vi "DHE_DRV_set_expdelay.vi"(7 "delay(ms)":sgl, 11 "error in (no error)":errorcluster) -> (15 "error out":errorcluster)   [LabVIEW 2016]
doc: "This VI closes the I/O interface with the instrument."
uses:
  c/lib/libarcDHE.so
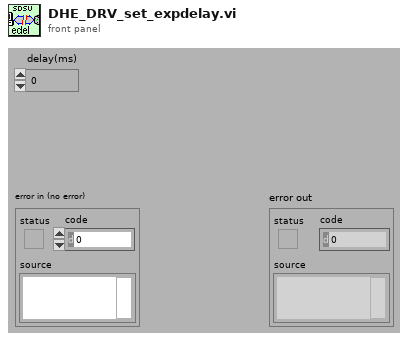
[diagram p1: front panel]
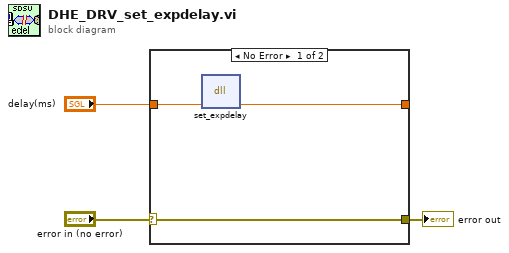
[diagram p0: block diagram]
diagram:
  n1 = case shown="No Error" "error in (no error)" {
    selector: "error in (no error)" -> [w4 w7]
    tunnel: "delay(ms)" -> [w6 w8]
    tunnel: [w4 w7] -> w2
    tunnel: [w5 w8] -> _
    frame No Error {
      n2 = dll-call lib="home/simager/panview/PAN/Modules/SDSU/private/c/lib/libarcDHE.so" fn="set_expdelay"("delay"=w6) -> ("delay"=w5:sgl)  [unwired: 3 in, 3 out]
    }
    frame Error {
    }
  }
  "error out" <- w2
